vi "solar_cfg Read (Ref).vi"(0 "Config Refnum":refnum<data-value>, 1 "Section":string, 2 "Comments (Key,Comment)":cluster{"Key":string, "Comment":string}[](array[cluster]), 5 "Key_Prefix (\"\")":string, 7 "Ctrl Refnum":refnum<vi>, 9 "Update Ctrl Value? (T)":bool=TRUE, 11 "error in (no error)":errorcluster, 12 "ArrayDelimiters (1D,2D)":string[](array[string]), 13 "Write If Not Found? (T)":bool=TRUE) -> (4 "dup Config Refnum":refnum<data-value>, 6 "Ctrl Value":variant, 10 "Found?":bool, 15 "error out":errorcluster)   [LabVIEW 2018]
doc: "Reads the values associated with a control reference from a specified section in a configuration file. If the Key is empty the control reference label is used instead. Set a Comment (#...) to add a description after the key's value. Clusters use the element lables are their key names. Set Enum as Strings to True to use the string item of an enum.\n\nSupported Data Types: \nI8..EXT, Enum, Boolean, String, Path, VISA Reference, Timestamp\n1D & 2D Arrays and Clusters of the data types above.\n\n[Section]\nKey = \"Value\" #Comment"
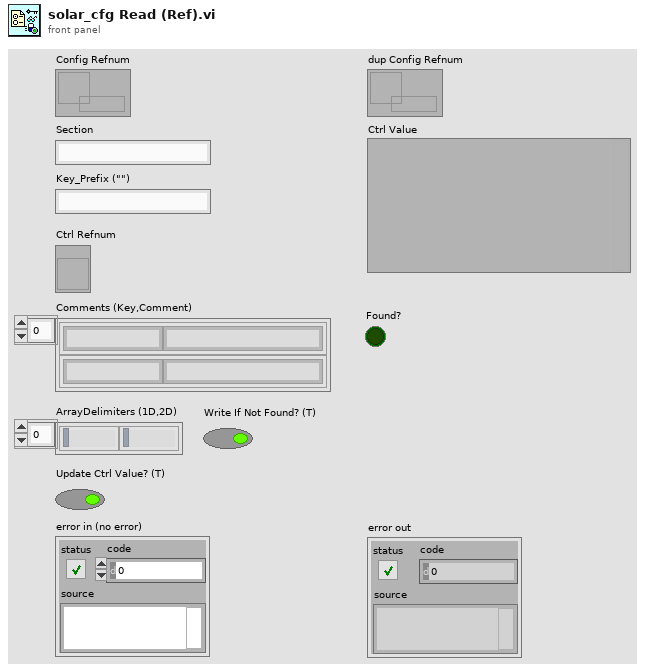
[diagram p1: front panel]
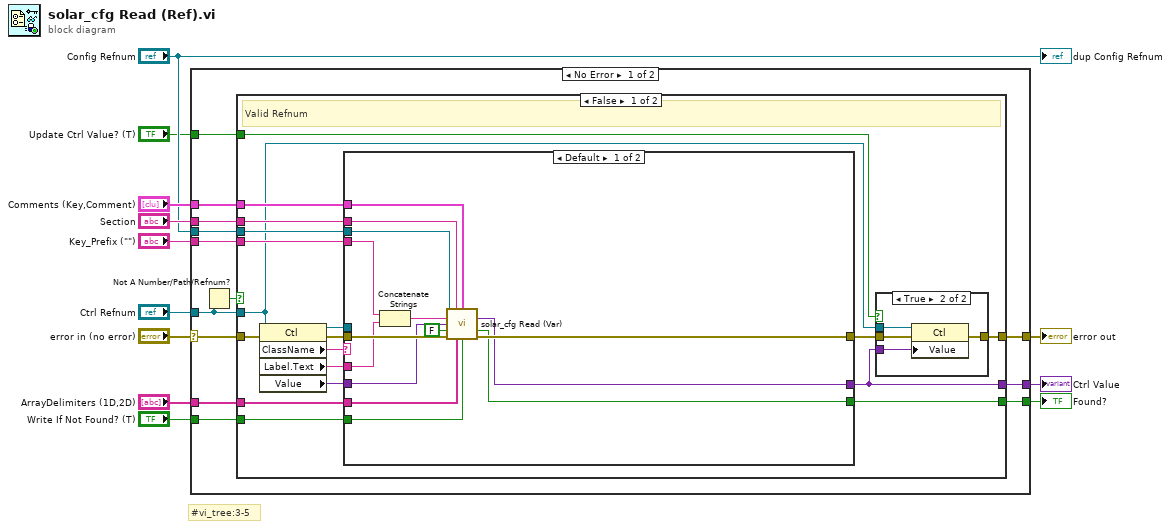
[diagram p0: block diagram]
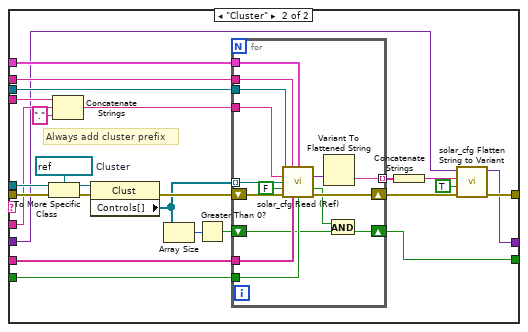
[diagram p2: hidden frame]
diagram:
  # "#vi_tree:3-5"
  n1 = case shown="No Error" "error in (no error)" {
    selector: "error in (no error)" -> [w25 w105]
    tunnel: "Key_Prefix (\"\")" -> [w24 _]
    tunnel: [w23 w105] -> w10
    tunnel: "Section" -> [w22 _]
    tunnel: [w15 _] -> w8
    tunnel: "Comments (Key,Comment)" -> [w21 _]
    tunnel: "ArrayDelimiters (1D,2D)" -> [w20 _]
    tunnel: "Write If Not Found? (T)" -> [w19 _]
    tunnel: "Ctrl Refnum" -> [w18 _]
    tunnel: "Config Refnum" -> [w17 _]
    tunnel: [w14 _] -> w2
    tunnel: "Update Ctrl Value? (T)" -> [w13 _]
    frame No Error {
      n2 = Not A Number/Path/Refnum?(number/path/refnum=w18) -> (NaN/Path/Refnum?=w16:bool)
      n3 = case "Invalid Refnum?" shown="False" w16 {
        tunnel: w25 -> [w34 w104]
        tunnel: w18 -> [w32 _]
        tunnel: [w43 w104] -> w23
        tunnel: w24 -> [w36 _]
        tunnel: w17 -> [w42 _]
        tunnel: [w41 _] -> w15
        tunnel: w22 -> [w40 _]
        tunnel: w20 -> [w39 _]
        tunnel: w21 -> [w38 _]
        tunnel: w19 -> [w37 _]
        tunnel: [w27 _] -> w14
        tunnel: w13 -> [w26 _]
        frame False {
          # "Valid Refnum"
          n4 = property class="Ctl"(reference=w32, error in=w34) -> (reference out=w28:refnum<vi>, error out=w33:errorcluster, "ClassName"=w31:string, "Label.Text"=w30:string, "Value"=w29:variant)
          n5 = case shown="Default" w31 {
            tunnel: w42 -> [w56 w71]
            tunnel: [w44 w58] -> w41
            tunnel: w40 -> [w53 w70]
            tunnel: w39 -> [w46 w64]
            tunnel: w38 -> [w52 w69]
            tunnel: w37 -> [w45 w63]
            tunnel: w36 -> [w48 w72]
            tunnel: w33 -> [w57 w80]
            tunnel: [w50 w75] -> w27
            tunnel: [w51 w76] -> w35
            tunnel: w30 -> [w55 w67]
            tunnel: w29 -> [w54 w65]
            tunnel: w28 -> [_ w79]
            frame Default {
              n6 = Concatenate Strings(w48, w55) -> (w49:string)
              n7 = call "solar_cfg Read (Var).vi"("Config Refnum"=w56, "Section"=w53, "Comments (Key,Comment)"=w52, "Key (\"\")"=w49, "Variant in"=w54, "Include Variant Name? (F)"=FALSE, "error in (no error)"=w57, "ArrayDelimiters (1D,2D)"=w46, "Write If Not Found? (T)"=w45) -> ("Variant out"=w50:variant, "Found?"=w44:bool, "error out"=w51:errorcluster)  [unwired: 3 in, 1 out]
            }
            frame "Cluster" {
              w82 = refnum<vi> refnum  # Cluster
              # "Always add cluster prefix"
              n8 = To More Specific Class(target class=w82, reference=w79, error in=w80) -> (specific class reference=w83:refnum<vi>, error out=w81:errorcluster)
              n9 = Concatenate Strings(w72, w67, "." ("string")) -> (w68:string)
              n10 = property class="Clust"(reference=w83, error in=w81) -> (error out=w74:errorcluster, "Controls[]"=w61:refnum<vi>[])  [unwired: 1 out]
              n11 = Array Size(array=w61) -> (size(s)=w60:i32)
              n12 = Greater Than 0?(x=w60) -> (x > 0?=w59:bool)
              n13 = for {
                tunnel: w71 -> [w96]
                tunnel: w70 -> [w95]
                tunnel: w69 -> [w94]
                tunnel: w68 -> [w93]
                tunnel: w61 -> [w91] mode=indexing
                shift-right: [w97] -> w73
                shift-left: w74 -> [w98]
                tunnel: w64 -> [w90]
                tunnel: w63 -> [w89]
                tunnel: [w87] -> w62 mode=indexing
                shift-right: [w84] -> w58
                shift-left: w59 -> [w86]
                n14 = call "solar_cfg Read (Ref).vi"("Config Refnum"=w96, "Section"=w95, "Comments (Key,Comment)"=w94, "Key_Prefix (\"\")"=w93, "Ctrl Refnum"=w91, "Update Ctrl Value? (T)"=FALSE, "error in (no error)"=w98, "ArrayDelimiters (1D,2D)"=w90, "Write If Not Found? (T)"=w89) -> ("Ctrl Value"=w88:variant, "Found?"=w85:bool, "error out"=w97:errorcluster)  [unwired: 3 in, 1 out]
                n15 = Variant To Flattened String(Variant=w88) -> (data string=w87:string)  [unwired: 1 out]
                n16 = And(x=w85, y=w86) -> (x .and. y?=w84:bool)
              }
              n17 = Concatenate Strings(w62) -> (w77:string)
              n18 = call "solar_cfg Flatten String to Variant.vi"("error in (no error)"=w73, "Keep Attributes? (F)"=TRUE, "Data String"=w77, "Variant in"=w65) -> ("error out"=w76:errorcluster, "Variant out"=w75:variant)  [unwired: 5 in, 1 out]
            }
          }
          n19 = case shown="True" w26 {
            tunnel: [w99 w103] -> w43
            tunnel: w35 -> [w99 w102]
            tunnel: w32 -> [_ w101]
            tunnel: w27 -> [_ w100]
            frame False {
              # "Do not update"
            }
            frame True {
              n20 = property class="Ctl"(reference=w101, error in=w102, "Value"=w100) -> (error out=w103:errorcluster)  [unwired: 1 out]
            }
          }
        }
        frame True {
          # "Invalid Refnum"
        }
      }
    }
    frame Error {
    }
  }
  "error out" <- w10
  "Found?" <- w8
  "Ctrl Value" <- w2
  "dup Config Refnum" <- "Config Refnum"
